vi "Get Trace Log.vi"(11 "Processing in":refnum<class "Processing.lvclass">) -> (2 "Trace Log":refnum<class "RequestTraceLog.lvclass">, 3 "Processing out":refnum<class "Processing.lvclass">)   [LabVIEW 2020, in "HTTP Server.lvlib" / "Processing.lvclass"]
uses:
  Processing.lvclass
  RequestTraceLog/RequestTraceLog.lvclass
  Processing.lvclass/Processing.ctl
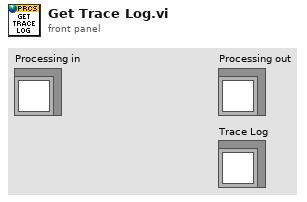
[diagram p1: front panel]
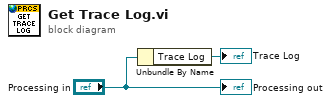
[diagram p0: block diagram]
diagram:
  n1 = Unbundle By Name("Processing in") -> ("Trace Log"=→"Trace Log":refnum<class "RequestTraceLog.lvclass">)
  "Processing out" <- "Processing in"
